vi "CallPPL.vi"(11 "Error in":errorcluster caption="Error in (no error)") -> (15 "Error out":errorcluster)   [LabVIEW 2019]
doc: "<Developer>\nGPower\n22/9 2019"
uses:
  <vilib>/GPower/Logger/Library/Logger Class/Logger/Severity Level.ctl
  <vilib>/GPower/Actor/Library/Actor Interface Class/Actor Interface.lvclass
  <vilib>/GPower/Logger - MCL/Library/MCL Logger Class/MCL Logger.lvclass
  C:/Program Files (x86)/National Instruments/LabVIEW 2019/vi.lib/GPower/Logger/Library/Logger Class/Logger.lvclass
  <vilib>/GPower/LVFile/Library/NewLVFile/NewLVFileByPath.vi
  <vilib>/GPower/AppControl/Library/Dynamic VI Control/OpenAndRun/OAR By Path.vi
  <vilib>/GPower/LVFile/Library/LVFileClass/LVFile/LVFile.lvclass
  <vilib>/GPower/LVFile/GPLVFile.lvlib
  <vilib>/GPower/AppControl/Library/GPAppControl.lvlib
  <vilib>/GPower/Message/Library/Message Class/Message.lvclass
  <vilib>/GPower/Logger/Library/Logger Class/Logger.lvclass
panel:
  in  "Boolean":bool
  in  "Multicolumn Listbox":i32(listbox)
  in  "PPL":i32(listbox)
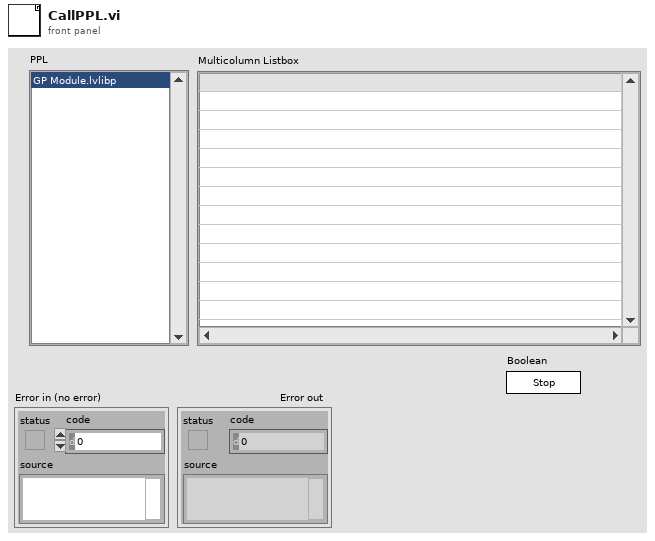
[diagram p1: front panel]
types:
  T1 = typedef "GP Logger.lvlib/Logger.lvclass/Severity Level.ctl" = enum16{"Emergency", "Alert", "Critical", "Error", "Warning", "Notice", "Info", "Debug"}
  T2 = typedef "GP Actor.lvlib/Actor Interface.lvclass/Registered Actor Events.ctl" = cluster{"Actor Messages":refnum<event-registration>, "Actor Stopped":refnum<event-registration>, "Actor Stop":refnum<event-registration>}
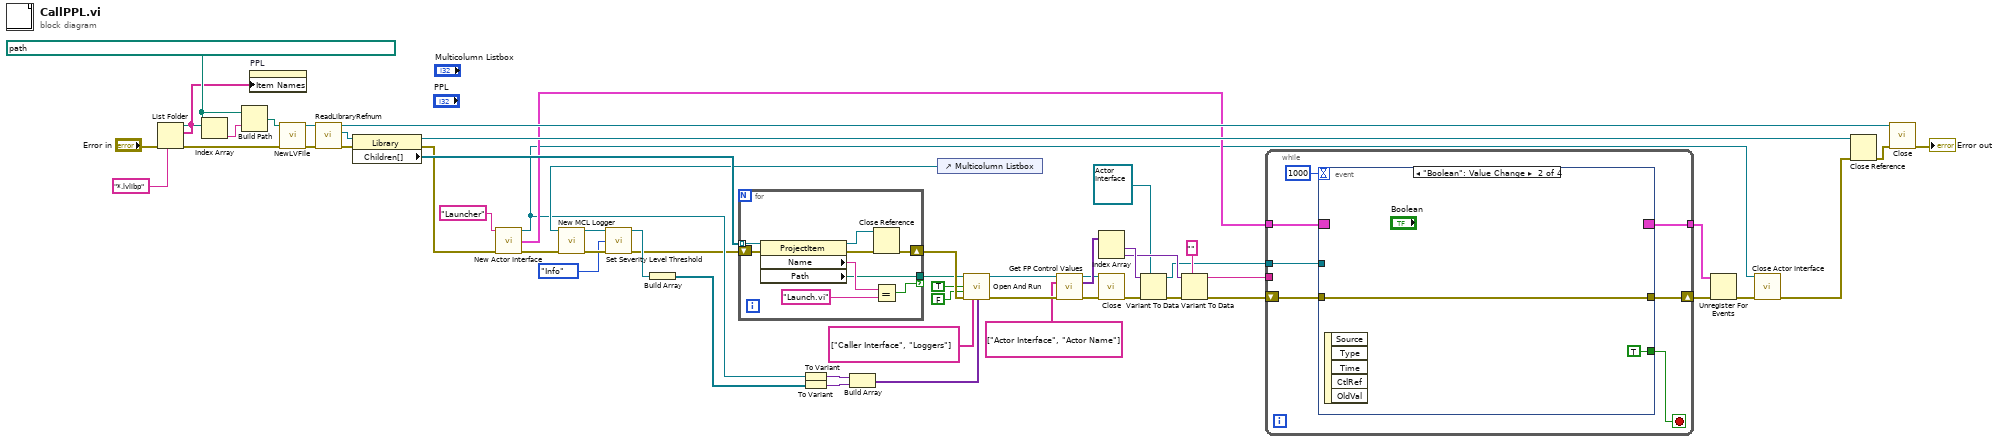
[diagram p0: block diagram]
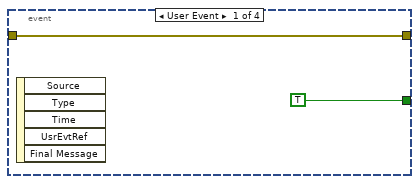
[diagram p2: hidden frame]
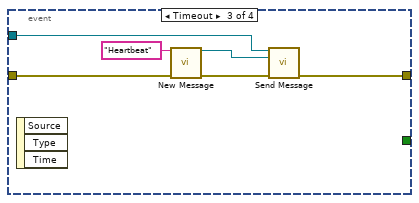
[diagram p3: hidden frame]
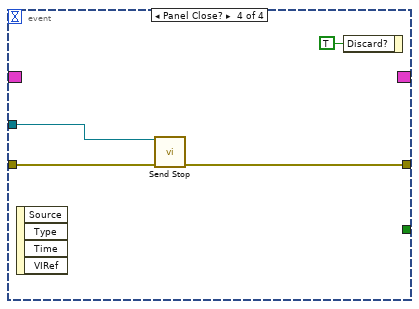
[diagram p4: hidden frame]
diagram:
  w53 = path "C:/Users/Kåre Juul Kirkegaard/Documents/github/Sandbox/PackProjectLibrary/Builds" ("path")
  n1 = List Folder(path=w53, pattern="*.lvlibp", error in="Error in") -> (filenames=w52:string[], error out=w49:errorcluster)  [unwired: 1 in, 2 out]
  n2 = Index Array(array=w52) -> (element=w51:string)  [unwired: 1 in]
  n3 = Build Path(base path=w53, name or relative path=w51) -> (appended path=w50:path)
  n4 = property on="PPL" class="LstBox (strict)"("Item Names"=w52) -> ()  [unwired: 2 in, 2 out]
  n5 = call-poly <vilib>:"NewLVFile.vi"("LV File Path"=w50, "Error in"=w49) -> ("New LV File Object"=w47:refnum<class "LVFile.lvclass">, "Error out"=w48:errorcluster)  [unwired: 12 in]
  n6 = call <vilib>:"ReadLibraryRefnum.vi"("Error in"=w48, "LV File Object in"=w47) -> ("Error out"=w43:errorcluster, "Library Reference"=w46:refnum<vi>, "LV File Object out"=w44:refnum<class "LVFile.lvclass">)  [unwired: 7 in]
  n7 = property class="Library"(reference=w46, error in=w43) -> (reference out=w41:refnum<vi>, error out=w15:errorcluster, "Children[]"=w40:refnum<vi>[])
  n8 = call <vilib>:"New Actor Interface.vi"("My Name"="Launcher", "Error in"=w15) -> ("New Actor Interface"=w20:refnum<class "Actor Interface.lvclass">, "Registered Actor Events"=w35:T2, "Error out"=w37:errorcluster)  [unwired: 11 in]
  n9 = To Variant(anything=w20) -> (Variant=w18:variant)
  n10 = control-ref of="Multicolumn Listbox"() -> (w38:refnum<vi>)
  n11 = call <vilib>:"New MCL Logger.vi"("Multicolumn Listbox"=w38, "Error in"=w37) -> ("MCL Logger"=w28:refnum<class "MCL Logger.lvclass">, "Error out"=w26:errorcluster)  [unwired: 12 in]
  n12 = call <vilib>:"Set Severity Level Threshold.vi"("Logger in"=w28, "Severity Level Threshold"=Severity_Level."Info", "Error in"=w26) -> ("Logger out"=w27:refnum<class "MCL Logger.lvclass">, "Error out"=w14:errorcluster)  [unwired: 11 in]
  n13 = Build Array(w27) -> (w19:refnum<class "MCL Logger.lvclass">[])
  n14 = for {
    tunnel: w40 -> [w61] mode=indexing
    shift-right: [w60] -> w23
    shift-left: w14 -> [w64]
    tunnel: [w57] -> w22 if=w56
    n15 = property class="ProjectItem"(reference=w61, error in=w64) -> (reference out=w63:refnum<vi>, error out=w62:errorcluster, "Name"=w59:string, "Path"=w57:path)
    n16 = Close Reference(reference=w63, error in (no error)=w62) -> (error out=w60:errorcluster)
    n17 = Equal?(x=w59, y="Launch.vi") -> (x = y?=w56:bool)
  }
  n18 = To Variant(anything=w19) -> (Variant=w17:variant)
  n19 = Build Array(w18, w17) -> (w16:variant[])
  n20 = call-poly <vilib>:"Open And Run.vi"("VI Path"=w22, "Wait Until VI Done?"=TRUE, "Transfer Refnum Ownership?"=FALSE, "Error in"=w23, "Control Names"=string[] ["Caller Interface", "Loggers"], "Control Values"=w16) -> ("New VI Refnum"=w30:refnum<vi>, "Error out"=w13:errorcluster)  [unwired: 7 in, 1 out]
  n21 = call <vilib>:"Get FP Control Values.vi"("VI Refnum in"=w30, "Control Names"=string[] ["Actor Interface", "Actor Name"], "Error in"=w13) -> ("VI Refnum out"=w29:refnum<vi>, "Control Values"=w39:variant[], "Error out"=w24:errorcluster)  [unwired: 10 in]
  n22 = Index Array(array=w39) -> (element #1=w11:variant, element #2=w10:variant)  [unwired: 2 in]
  n23 = call <vilib>:"Close.vi"("VI Refnum"=w29, "Error in"=w24) -> ("Error out"=w6:errorcluster)  [unwired: 10 in, 3 out]
  n24 = Variant To Data(error in=w6, type=refnum<class "Actor Interface.lvclass"> refnum ("New Actor Interface"), Variant=w11) -> (data=w7:refnum<class "Actor Interface.lvclass">, error out=w5:errorcluster)
  n25 = Variant To Data(error in=w5, type="", Variant=w10) -> (data=w3:string, error out=w4:errorcluster)
  n26 = while {
    tunnel: w35 -> [w71]
    shift-right: [w68] -> w34
    shift-left: w4 -> [w69]
    tunnel: [w67] -> w32
    tunnel: w7 -> [w66]
    tunnel: w3 -> [_]
    stop <- w70 stop-if-true
    n27 = event shown="[1] \"Boolean\": Value Change" {
      selector: w71 -> [_ _ _ _]
      dyn-events: [_ _ _ _] -> w67
      timeout: 1000 -> [_ _ _ _]
      tunnel: [TRUE TRUE _ _] -> w70
      tunnel: w69 -> [w72 w74 w81 w84]
      tunnel: [w72 w74 w79 w82] -> w68
      tunnel: w66 -> [_ _ w76 w83]
      event User Event {
        n28 = event-data() -> ()  [unwired: 1 in, 5 out]
      }
      event "Boolean": Value Change {
        n29 = event-data() -> ()  [unwired: 1 in, 5 out]
      }
      event Timeout {
        n30 = event-data() -> ()  [unwired: 1 in, 3 out]
        n31 = call <vilib>:"New Message.vi"("Name"="Heartbeat", "Error in"=w81) -> ("New Message"=w77:refnum<class "Message.lvclass">, "Error out"=w80:errorcluster)  [unwired: 12 in]
        n32 = call <vilib>:"Send Message.vi"("Receiver"=w76, "Message"=w77, "error in (no error)"=w80) -> ("error out"=w79:errorcluster)  [unwired: 12 in]
      }
      event Panel Close? {
        n33 = event-data() -> ()  [unwired: 1 in, 4 out]
        n34 = call <vilib>:"Send Stop.vi"("Receiver"=w83, "Error in"=w84) -> ("Error out"=w82:errorcluster)  [unwired: 13 in]
        n35 = event-data("Discard?"=TRUE) -> ()  [unwired: 1 in, 1 out]
      }
    }
  }
  n36 = Unregister For Events(event registration refnum=w32, error in=w34) -> (error out=w33:errorcluster)
  n37 = call <vilib>:"Close Actor Interface.vi"("Actor Interface"=w20, "Error in"=w33) -> ("Error out"=w31:errorcluster)  [unwired: 13 in]
  n38 = Close Reference(reference=w41, error in (no error)=w31) -> (error out=w42:errorcluster)
  n39 = call-dynamic <vilib>:"Close.vi"("LV File Object"=w44, "Error in"=w42) -> ("Error out"=→"Error out":errorcluster)  [unwired: 13 in]
